vi "Example Simple.vi"() -> ()   [LabVIEW 2010]
uses:
  C:/tf/play/labview/Tinkerforge.dll
  Tinkerforge.dll
panel:
  out "connectedBrickletUID":string
  out "connectedBrickletDeviceIdentifier":i32
  out "messagesFromBricklet":i64
  out "messagesFromBrick":i64
  in  "uid":string="cnq"
  in  "port":i32=4223
  in  "host":string="localhost"
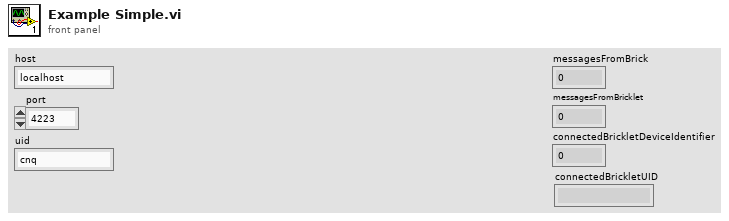
[diagram p1: front panel]
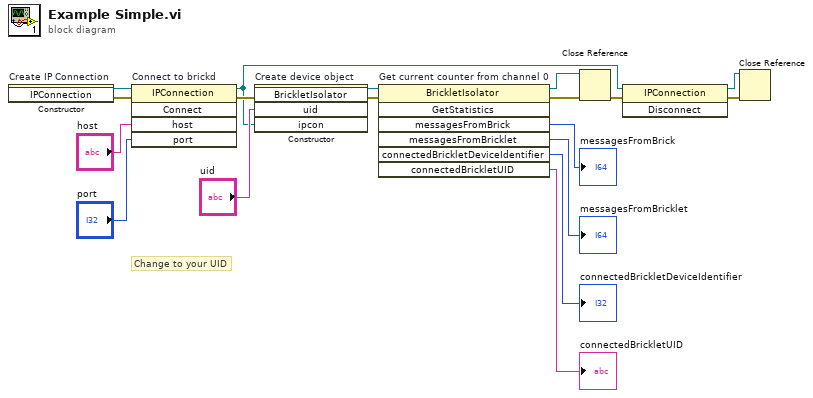
[diagram p0: block diagram]
diagram:
  # "Change to your UID"
  n1 = constructor on="Create IP Connection" class="IPConnection"() -> (reference out=w18:refnum<k24>, error out=w7:errorcluster)  [unwired: 3 in, 1 out]
  n2 = invoke on="Connect to brickd" class="IPConnection" method="Connect"(reference=w18, error in=w7, "host"="host", "port"="port") -> (reference out=w9:refnum<k24>, error out=w14:errorcluster)  [unwired: 1 in, 3 out]
  n3 = constructor on="Create device object" class="BrickletIsolator"(error in=w14, "uid"="uid", "ipcon"=w9) -> (reference out=w12:refnum<k24>, error out=w13:errorcluster)  [unwired: 2 in, 3 out]
  n4 = invoke on="Get current counter from channel 0" class="BrickletIsolator" method="GetStatistics"(reference=w12, error in=w13) -> (reference out=w5:refnum<k24>, error out=w6:errorcluster, "messagesFromBrick"=→"messagesFromBrick":i64, "messagesFromBricklet"=→"messagesFromBricklet":i64, "connectedBrickletDeviceIdentifier"=→"connectedBrickletDeviceIdentifier":i32, "connectedBrickletUID"=→"connectedBrickletUID":string)  [unwired: 5 in, 1 out]
  n5 = Close Reference(reference=w5, error in (no error)=w6) -> (error out=w11:errorcluster)
  n6 = invoke class="IPConnection" method="Disconnect"(reference=w9, error in=w11) -> (reference out=w8:refnum<k24>, error out=w10:errorcluster)  [unwired: 1 in, 1 out]
  n7 = Close Reference(reference=w8, error in (no error)=w10) -> ()  [unwired: 1 out]
